vi "readTemperature.vi"(8 "error in (no error)":errorcluster, 10 "ElectrometerController in":refnum<class "ElectrometerController.lvclass">, 11 "ElectrometerState in":refnum<class "ElectrometerState.lvclass">) -> (0 "error out":errorcluster, 2 "ElectrometerController out":refnum<class "ElectrometerController.lvclass">, 3 "ElectrometerState out":refnum<class "ElectrometerState.lvclass">)   [LabVIEW 2016, in "ElectrometerState.lvclass"]
uses:
  ElectrometerState.lvclass
  ElectrometerController/ElectrometerController.lvclass
  Electrometer.lvclass
  ElectrometerConfiguration/ElectrometerInternalConfiguration.lvclass
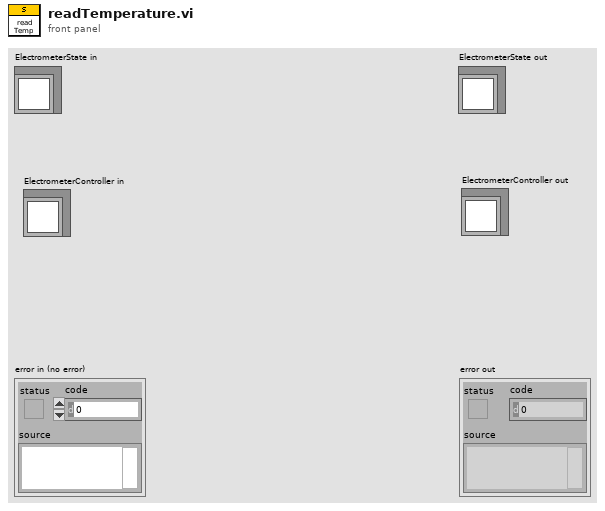
[diagram p1: front panel]
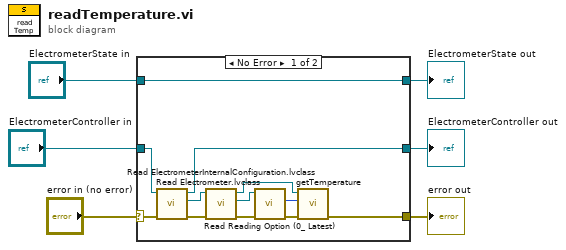
[diagram p0: block diagram]
diagram:
  n1 = case shown="No Error" "error in (no error)" {
    selector: "error in (no error)" -> [w16 w21]
    tunnel: [w15 w21] -> w5
    tunnel: [w18 w20] -> w3
    tunnel: "ElectrometerState in" -> [w18 w20]
    tunnel: "ElectrometerController in" -> [w17 w19]
    tunnel: [w7 w19] -> w1
    frame No Error {
      n2 = call-dynamic "Read Electrometer.lvclass.vi"("error in (no error)"=w16, "ElectrometerController in"=w17) -> ("error out"=w13:errorcluster, "Electrometer.lvclass"=w14:refnum<class "Electrometer.lvclass">, "ElectrometerController out"=w7:refnum<class "ElectrometerController.lvclass">)  [unwired: 7 in]
      n3 = call-dynamic "Read ElectrometerInternalConfiguration.lvclass.vi"("error in (no error)"=w13, "Electrometer in"=w14) -> ("error out"=w11:errorcluster, "ElectrometerInternalConfiguration.lvclass"=w12:refnum<class "ElectrometerInternalConfiguration.lvclass">, "Electrometer out"=w8:refnum<class "Electrometer.lvclass">)  [unwired: 7 in]
      n4 = call-dynamic "Read Reading Option (0_ Latest).vi"("error in (no error)"=w11, "ElectrometerInternalConfiguration in"=w12) -> ("error out"=w10:errorcluster, "Reading Option (0: Latest)"=w9:i32)  [unwired: 7 in, 1 out]
      n5 = call "getTemperature.vi"("error in (no error)"=w10, "Reading Option (0: Latest)"=w9, "Electrometer in"=w8) -> ("error out"=w15:errorcluster)  [unwired: 6 in, 2 out]
    }
    frame Error {
    }
  }
  "error out" <- w5
  "ElectrometerState out" <- w3
  "ElectrometerController out" <- w1
